vi "runPythonServer.vi"() -> ()   [LabVIEW 2018]
panel:
  in  "error in (no error)":errorcluster
  out "error out":errorcluster
  in  "command line (built-in)":string="C:/Users/adminKnorr/.conda/envs/yoloEnv/python.exe C:\\Users\\adminKnorr\\Documents\\David\\Github\\PyLV_TCP_1.2\\serverTCP.py"
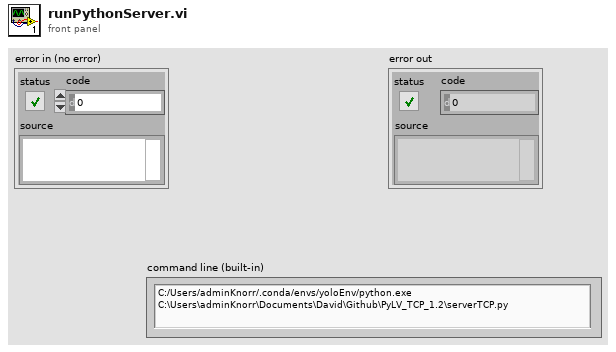
[diagram p1: front panel]
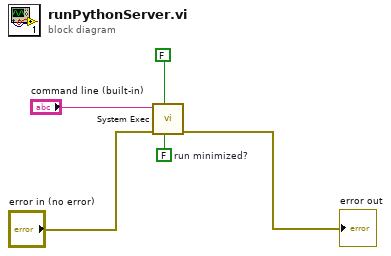
[diagram p0: block diagram]
diagram:
  w4 = FALSE  # run minimized?
  n1 = call <vilib>:"System Exec.vi"("run minimized? (F)"=w4, "wait until completion? (T)"=FALSE, "error in (no error)"="error in (no error)", "command line"="command line (built-in)") -> ("error out"=→"error out":errorcluster)  [unwired: 2 in, 5 out]
